vi "ini_sesion.vi"(8 "error in (no error)":errorcluster, 11 "5785_2_X_400MHz_Rx_as_scop in":refnum<class "5785_2_X_400MHz_Rx_as_scop.lvclass">) -> (0 "error out":errorcluster, 3 "5785_2_X_400MHz_Rx_as_scop out":refnum<class "5785_2_X_400MHz_Rx_as_scop.lvclass">)   [LabVIEW 2021, in "5785_2_X_400MHz_Rx_as_scop.lvclass"]
uses:
  5785_2_X_400MHz_Rx_as_scop.lvclass
  5785_2_X_400MHz_Rx_as_scop.lvclass/5785_2_X_400MHz_Rx_as_scop.ctl
  <instrlib>/FlexRIO/API/Host/v1/NI FlexRIO/API/Reference Clock Source.ctl
  <vilib>/FPGAPlugInAG/PXIe-5785 (KU060)/niLvFpga_Open_PXIe-5785 (KU060).vi
  <vilib>/rvi/interface/common/dynamic/niFpgaDynamicAddResources.vi
  <instrlib>/FlexRIO/API/Host/v1/NI FlexRIO/API/Configure Reference Clock.vi
  <vilib>/Utility/error.llb/Error Cluster From Error Code.vi
  <vilib>/rvi/interface/common/niFpgaWaitOnOcc.vi
  <instrlib>/FlexRIO/API/Host/v1/NI FlexRIO/API/Get Property Reference - Fpga Small.vi
  <vilib>/rvi/errors/niLvFpgaAdjustHostInterfaceError.vi
  <vilib>/rvi/interface/nirviOpenFPGA/nirviOpenFPGA.xnode
  FPGA Bitfiles/5785_IQ_gen_2_x_400MHz_transfer_back.lvbitx
  <vilib>/rvi/interface/nirviMethod/nirviMethod.xnode
  <vilib>/rvi/interface/nirviReadWriteControl/nirviReadWriteControl.xnode
  <instrlib>/FlexRIO/API/Host/v1/NI FlexRIO API v1.lvlib
  <resource>/objmgr/niflexrioapiStream.rc
  <resource>/objmgr/niflexrioapi.rc
  <vilib>/FPGAPlugInAG/Dynamic/niLvFpga_ConfigureFifo_Dynamic.vi
  <vilib>/rvi/errors/niLvFpgaMergeErrorWithErrorCode.vi
  <resource>/objmgr/niflexrioapiChannel.rc
  <vilib>/FPGAPlugInAG/Dynamic/niLvFpga_StopFifo_Dynamic.vi
  <vilib>/FPGAPlugInAG/Dynamic/niLvFpga_StartFifo_Dynamic.vi
  NiFpgaLv.dll
  <vilib>/rvi/interface/Simulation/niFpgaSimulationCallBeginRW.vi
panel:
  out "Actual Depth":u32
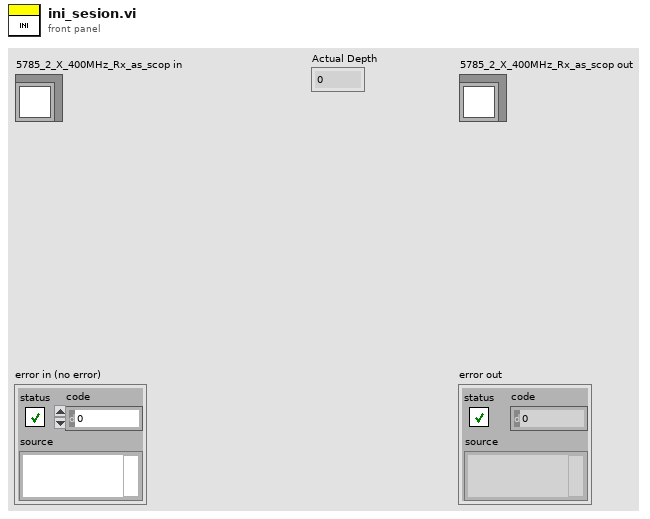
[diagram p1: front panel]
types:
  T1 = typedef "nirio_resource_hc.ctl" = tag
  T2 = typedef "NI FlexRIO API v1.lvlib/Reference Clock Source.ctl" = i32
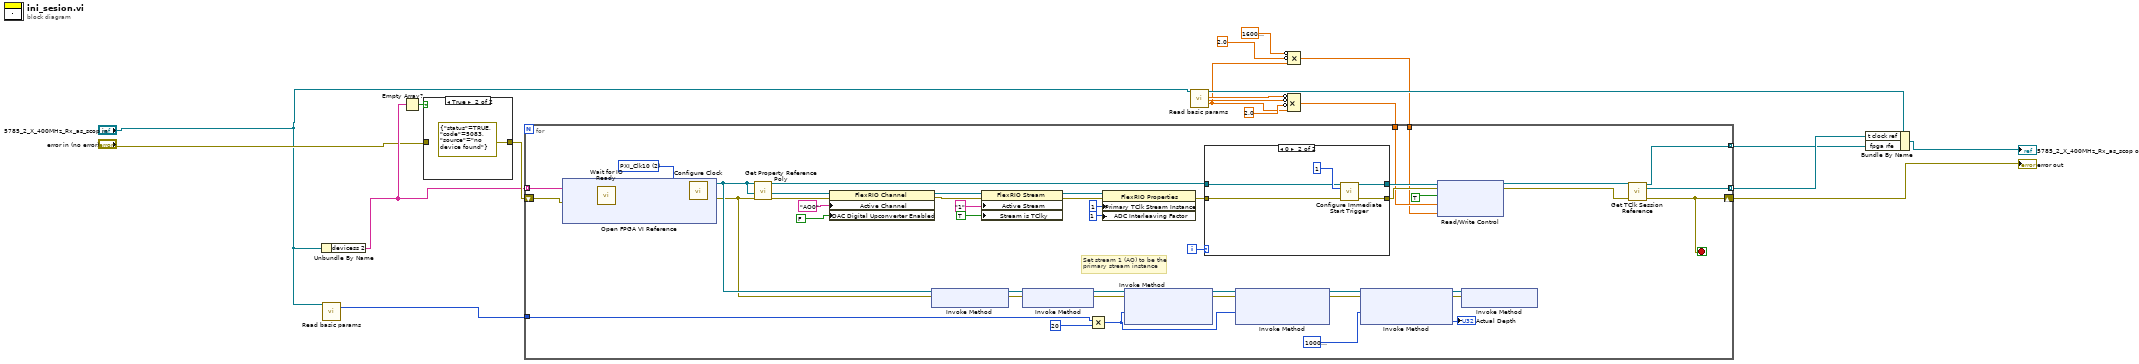
[diagram p0: block diagram]
diagram:
  n1 = Unbundle By Name("5785_2_X_400MHz_Rx_as_scop in") -> ("devicess 2"=w15:T1[])
  n2 = call-dynamic "Read basic params.vi"("device_type in"="5785_2_X_400MHz_Rx_as_scop in") -> ("buffer size"=w16:u32)  [unwired: 13 in, 5 out]
  n3 = Empty Array?(array=w15) -> (empty?=w18:bool)
  n4 = case shown="True" w18 {
    tunnel: [w20 errorcluster {"status"=TRUE, "code"=5083, "source"="no device found"} ("error in (no error)")] -> w17
    tunnel: "error in (no error)" -> [w20 _]
    frame False {
    }
    frame True {
    }
  }
  n5 = call-dynamic "Read basic params.vi"("device_type in"="5785_2_X_400MHz_Rx_as_scop in") -> ("device_type out"=w9:refnum<class "5785_2_X_400MHz_Rx_as_scop.lvclass">, "Fs  FPGA"=w8:dbl, "SPC"=w7:dbl, "center frequency (Hz)"=w4:dbl)  [unwired: 13 in, 2 out]
  n6 = Compound Arithmetic op=MULTIPLY(invert w8, invert w7, invert 2.0 ("value"), w4) -> (w5:dbl)
  n7 = Compound Arithmetic op=MULTIPLY(invert 1600000000.0 ("value"), invert 2.0 ("value"), w4) -> (w1:dbl)
  n8 = for {
    shift-right: [w46] -> w11
    shift-left: w17 -> [w61]
    tunnel: [w34] -> w19 mode=indexing
    tunnel: w15 -> [w50] mode=indexing
    tunnel: w16 -> [w36]
    tunnel: [w33] -> w14 mode=indexing
    tunnel: w5 -> [w32]
    tunnel: w1 -> [w31]
    i -> [w64]
    stop <- w46 stop-if-true
    w49 = T2 2 items=["Default", "Onboard", "PXI_Clk10", "External", "None", "Baseboard Reference"] ("reference clock source")
    # "Set stream 1 (AO) to be the\nprimary stream instance"
    n9 = xnode "Open FPGA VI Reference"("error in"=w61, "resource name"=w50) -> ("FPGA VI Reference Out"=w63:refnum<k20>, "error out"=w62:errorcluster)
    n10 = call <instrlib>:"Wait for IO Ready.vi"("fpga interface in"=w63, "error in"=w62) -> ("fpga interface out"=w48:refnum<k20>, "error out"=w47:errorcluster)  [unwired: 10 in, 2 out]
    n11 = call-poly <instrlib>:"Configure Clock.vi"("fpga interface in"=w48, "reference clock source"=w49, "error in"=w47) -> ("fpga interface out"=w42:refnum<k20>, "error out"=w41:errorcluster)  [unwired: 11 in]
    n12 = call-poly <instrlib>:"Get Property Reference Poly.vi"("error in (no error)"=w41, "fpga interface in"=w42) -> ("error out"=w53:errorcluster, "property reference"=w54:refnum<k20>)  [unwired: 4 in, 1 out]
    n13 = property class="FlexRIO Channel"(reference=w54, error in=w53, "Active Channel"="AO0", "DAC Digital Upconverter Enabled"=FALSE ("Analog Output:DAC Digital Upconverter Enabled")) -> (reference out=w52:refnum<k20>, error out=w51:errorcluster)
    n14 = xnode "Invoke Method"("FPGA VI Reference In"=w42, "error in"=w41) -> ("FPGA VI Reference Out"=w39:refnum<k20>, "error out"=w40:errorcluster)
    n15 = property class="FlexRIO Stream"(reference=w52, error in=w51, "Active Stream"="1", "Stream is TClky"=TRUE ("Configuration:Stream is TClky")) -> (reference out=w68:refnum<k20>, error out=w67:errorcluster)
    n16 = xnode "Invoke Method"("FPGA VI Reference In"=w39, "error in"=w40) -> ("FPGA VI Reference Out"=w37:refnum<k20>, "error out"=w38:errorcluster)
    n17 = Multiply(x=w36, y=u32 20) -> (x*y=w58:u32)
    n18 = property class="FlexRIO Properties"(reference=w68, error in=w67, "Primary TClk Stream Instance"=1 ("Device:Primary TClk Stream Instance"), "ADC Interleaving Factor"=1 ("Device:ADC:Interleaving Factor")) -> (error out=w65:errorcluster)  [unwired: 1 out]
    n19 = xnode "Invoke Method"("FPGA VI Reference In"=w37, "error in"=w38, "Requested Depth"=w58) -> ("FPGA VI Reference Out"=w60:refnum<k20>, "error out"=w59:errorcluster)  [unwired: 1 out]
    n20 = case shown="0" w64 {
      tunnel: w42 -> [w71 w75]
      tunnel: [w71 w74] -> w45
      tunnel: [w70 w73] -> w44
      tunnel: w65 -> [w70 w72]
      frame 1, Default {
      }
      frame 0 {
        n21 = call <instrlib>:"Configure Immediate Start Trigger.vi"("fpga interface in"=w75, "trigger instance"=u32 1, "error in"=w72) -> ("fpga interface out"=w74:refnum<k20>, "error out"=w73:errorcluster)  [unwired: 10 in, 1 out]
      }
    }
    n22 = xnode "Invoke Method"("FPGA VI Reference In"=w60, "error in"=w59, "Requested Depth"=w58) -> ("FPGA VI Reference Out"=w27:refnum<k20>, "error out"=w26:errorcluster)  [unwired: 1 out]
    n23 = xnode "Invoke Method"("FPGA VI Reference In"=w27, "error in"=w26, "Requested Depth"=u32 10000000) -> ("FPGA VI Reference Out"=w25:refnum<k20>, "error out"=w24:errorcluster, "Actual Depth"=→"Actual Depth":u32)
    n24 = xnode "Read/Write Control"("FPGA VI Reference In"=w45, "error in"=w44, "reset system clock"=TRUE, "frequency shift Tx"=w32, "frequency shift Rx"=w31) -> ("FPGA VI Reference Out"=w30:refnum<k20>, "error out"=w29:errorcluster)
    n25 = xnode "Invoke Method"("FPGA VI Reference In"=w25, "error in"=w24) -> ()  [unwired: 2 out]
    n26 = call <instrlib>:"Get TClk Session Reference.vi"("fpga interface in"=w30, "error in"=w29) -> ("fpga interface out"=w33:refnum<k20>, "tclk session reference"=w34:refnum<k20>, "error out"=w46:errorcluster)  [unwired: 11 in]
  }
  "error out" <- w11
  n27 = Bundle By Name(cluster=w9, "t clock ref"=w19, "fpga rfe"=w14) -> (→"5785_2_X_400MHz_Rx_as_scop out":refnum<class "5785_2_X_400MHz_Rx_as_scop.lvclass">)
